vi "RichToFlatnixnet_grpc_SetSubPropertyRequest.vi"(5 "OutputClusterType":T1, 11 "InputCluster":T4) -> (3 "OutputCluster":T1)   [LabVIEW 2025, in "grpc-xnet_client.lvlib"]
uses:
  grpc-xnet_client.lvlib
  nixnet_grpc_SetSubPropertyRequest.ctl
  nixnet_grpc_SetSubPropertyRequest_subproperty_id_enum/nixnet_grpc_SetSubPropertyRequest_subproperty_id_enum.lvclass
  nixnet_grpc_SetSubPropertyRequest_property_value/nixnet_grpc_SetSubPropertyRequest_property_value.lvclass
  nidevice_grpc_Session.ctl
  nixnet_grpc_SetSubPropertyRequest_Flat.ctl
  nidevice_grpc_Session_Flat.ctl
  nixnet_grpc_SubProperty.ctl
  nixnet_grpc_SetSubPropertyRequest_subproperty_id_enum/nixnet_grpc_SetSubPropertyRequest_subproperty_id_enum.lvclass/nixnet_grpc_SetSubPropertyRequest_subproperty_id_enum.ctl
  nixnet_grpc_SetSubPropertyRequest_property_value/nixnet_grpc_SetSubPropertyRequest_property_value.lvclass/nixnet_grpc_SetSubPropertyRequest_property_value.ctl
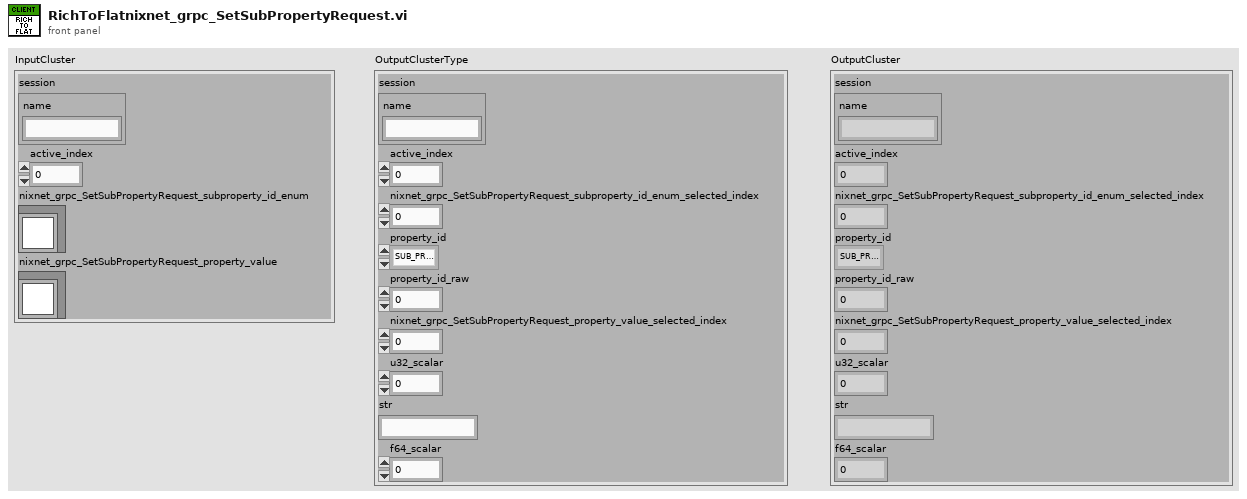
[diagram p1: front panel]
types:
  T1 = typedef "grpc-xnet_client.lvlib/nixnet_grpc_SetSubPropertyRequest_Flat.ctl" = cluster{"session":T2, "active_index":u32, "nixnet_grpc_SetSubPropertyRequest_subproperty_id_enum_selected_index":i32, "property_id":T3, "property_id_raw":u32, "nixnet_grpc_SetSubPropertyRequest_property_value_selected_index":i32, "u32_scalar":u32, "str":string, "f64_scalar":dbl}
  T2 = typedef "grpc-xnet_client.lvlib/nidevice_grpc_Session_Flat.ctl" = cluster{"name":string}
  T3 = typedef "grpc-xnet_client.lvlib/nixnet_grpc_SubProperty.ctl" = enum32{"SUB_PROPERTY_UNSPECIFIED", "SUB_PROPERTY_SESSION_SUB_CAN_START_TIME_OFF", "SUB_PROPERTY_SESSION_SUB_CAN_TX_TIME", "SUB_PROPERTY_SESSION_SUB_LIN_TX_N_CORRUPTED_CHKSUMS", "SUB_PROPERTY_SESSION_SUB_OUTPUT_QUEUE_UPDATE_FREQ", "SUB_PROPERTY_SESSION_SUB_J1939_ADDR_FILTER", "SUB_PROPERTY_SESSION_SUB_SKIP_N_CYCLIC_FRAMES"}
  T4 = typedef "grpc-xnet_client.lvlib/nixnet_grpc_SetSubPropertyRequest.ctl" = cluster{"session":T5, "active_index":u32, "nixnet_grpc_SetSubPropertyRequest_subproperty_id_enum":refnum<class "nixnet_grpc_SetSubPropertyRequest_subproperty_id_enum.lvclass">, "nixnet_grpc_SetSubPropertyRequest_property_value":refnum<class "nixnet_grpc_SetSubPropertyRequest_property_value.lvclass">}
  T5 = typedef "grpc-xnet_client.lvlib/nidevice_grpc_Session.ctl" = cluster{"name":string}
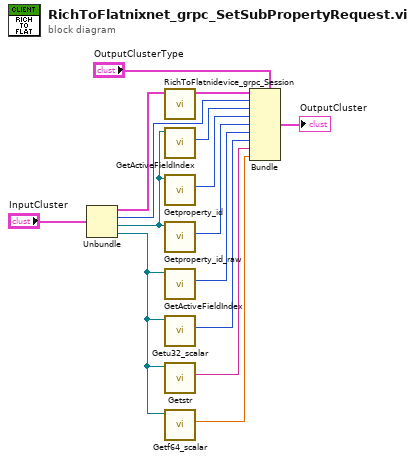
[diagram p0: block diagram]
diagram:
  n1 = Unbundle "Unbundle"("InputCluster") -> ("session"=w12:T5, "active_index"=w10:u32, "nixnet_grpc_SetSubPropertyRequest_subproperty_id_enum"=w9:refnum<class "nixnet_grpc_SetSubPropertyRequest_subproperty_id_enum.lvclass">, "nixnet_grpc_SetSubPropertyRequest_property_value"=w5:refnum<class "nixnet_grpc_SetSubPropertyRequest_property_value.lvclass">)
  n2 = call "RichToFlatnidevice_grpc_Session.vi"("InputCluster"=w12) -> ("OutputCluster"=w11:T2)  [unwired: 10 in]
  n3 = call "GetActiveFieldIndex.vi"("OneOfTemplate in"=w9) -> ("Active Field Index"=w8:i32)  [unwired: 8 in, 2 out]
  n4 = call "Getproperty_id.vi"("OneOfTemplate in"=w9) -> ("Get_Val"=w7:T3)  [unwired: 8 in, 2 out]
  n5 = call "Getproperty_id_raw.vi"("OneOfTemplate in"=w9) -> ("Get_Val"=w6:u32)  [unwired: 8 in, 2 out]
  n6 = call "GetActiveFieldIndex.vi"("OneOfTemplate in"=w5) -> ("Active Field Index"=w4:i32)  [unwired: 8 in, 2 out]
  n7 = call "Getu32_scalar.vi"("OneOfTemplate in"=w5) -> ("Get_Val"=w3:u32)  [unwired: 8 in, 2 out]
  n8 = call "Getstr.vi"("OneOfTemplate in"=w5) -> ("Get_Val"=w2:string)  [unwired: 8 in, 2 out]
  n9 = call "Getf64_scalar.vi"("OneOfTemplate in"=w5) -> ("Get_Val"=w1:dbl)  [unwired: 8 in, 2 out]
  n10 = Bundle "Bundle"(cluster="OutputClusterType", "session"=w11, "active_index"=w10, "nixnet_grpc_SetSubPropertyRequest_subproperty_id_enum_selected_index"=w8, "property_id"=w7, "property_id_raw"=w6, "nixnet_grpc_SetSubPropertyRequest_property_value_selected_index"=w4, "u32_scalar"=w3, "str"=w2, "f64_scalar"=w1) -> (→"OutputCluster":T1)
